vi "niDTS WLAN UTIL to Payload Length.vi"(9 "CH BW":T1, 10 "WLAN Type":T2) -> (2 "Payload Length":i32)   [LabVIEW 2015, in "niDTS WLAN.lvlib"]
uses:
  niDTS WLAN.lvlib
  Includes/niDTS WLAN INC Type.ctl
  Includes/niDTS WLAN INC CH BW.ctl
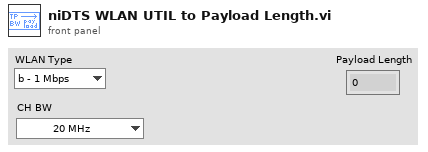
[diagram p1: front panel]
types:
  T1 = typedef "niDTS WLAN.lvlib/niDTS WLAN INC CH BW.ctl" = enum16{"20 MHz", "40 MHz", "80 MHz", "160 MHz"}
  T2 = typedef "niDTS WLAN.lvlib/niDTS WLAN INC Type.ctl" = enum16{"b - 1 Mbps", "b - 2 Mbps", "b - 5.5 Mbps", "b - 11 Mbps", "ag - 6 Mbps", "ag - 9 Mbps", "ag - 12 Mbps", "ag - 18 Mbps", "ag - 24 Mbps", "ag - 36 Mbps", "ag - 48 Mbps", "ag - 54 Mbps", "n - MCS0", "n - MCS1", "n - MCS2", "n - MCS3", "n - MCS4", "n - MCS5", "n - MCS6", "n - MCS7", "n - MCS8", "n - MCS9", "n - MCS10", "n - MCS11", "n - MCS12", "n - MCS13", "n - MCS14", "n - MCS15", "n - MCS16", "n - MCS17", "n - MCS18", "n - MCS19", "n - MCS20", "n - MCS21", "n - MCS22", "n - MCS23", "n - MCS24", "n - MCS25", "n - MCS26", "n - MCS27", "n - MCS28", "n - MCS29", "n - MCS30", "n - MCS31", "ac - MCS0 -1", "ac - MCS1 -1", "ac - MCS2 -1", "ac - MCS3 -1", "ac - MCS4 -1", "ac - MCS5 -1", "ac - MCS6 -1", "ac - MCS7 -1", "ac - MCS8 -1", "ac - MCS9 -1", "ac - MCS0 -2", "ac - MCS1 -2", "ac - MCS2 -2", "ac - MCS3 -2", "ac - MCS4 -2", "ac - MCS5 -2", "ac - MCS6 -2", "ac - MCS7 -2", "ac - MCS8 -2", "ac - MCS9 -2", "ac - MCS0 -3", "ac - MCS1 -3", "ac - MCS2 -3", "ac - MCS3 -3", "ac - MCS4 -3", "ac - MCS5 -3", "ac - MCS6 -3", "ac - MCS7 -3", "ac - MCS8 -3", "ac - MCS9 -3", "ac - MCS0 -4", "ac - MCS1 -4", "ac - MCS2 -4", "ac - MCS3 -4", "ac - MCS4 -4", "ac - MCS5 -4", "ac - MCS6 -4", "ac - MCS7 -4", "ac - MCS8 -4", "ac - MCS9 -4"}
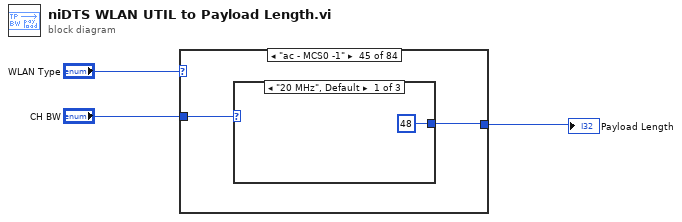
[diagram p0: block diagram]
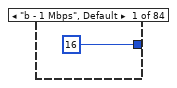
[diagram p2: hidden frame]
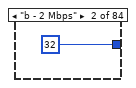
[diagram p3: hidden frame]
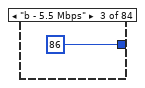
[diagram p4: hidden frame]
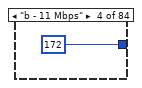
[diagram p5: hidden frame]
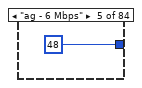
[diagram p6: hidden frame]
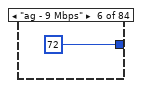
[diagram p7: hidden frame]
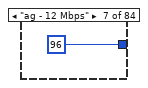
[diagram p8: hidden frame]
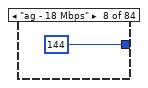
[diagram p9: hidden frame]
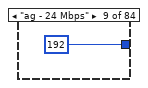
[diagram p10: hidden frame]
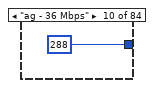
[diagram p11: hidden frame]
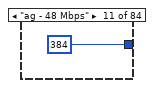
[diagram p12: hidden frame]
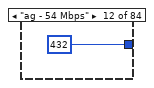
[diagram p13: hidden frame]
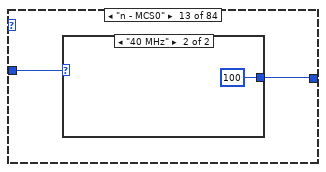
[diagram p14: hidden frame]
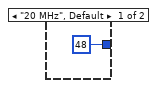
[diagram p15: hidden frame]
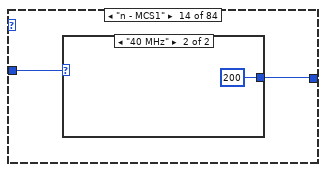
[diagram p16: hidden frame]
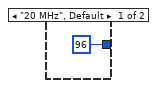
[diagram p17: hidden frame]
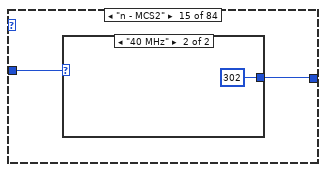
[diagram p18: hidden frame]
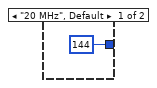
[diagram p19: hidden frame]
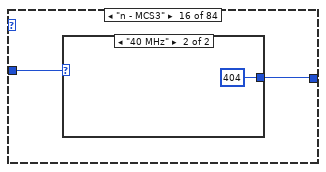
[diagram p20: hidden frame]
diagram:
  n1 = case shown="\"ac - MCS0 -1\"" "WLAN Type" {
    tunnel: [16 ("Payload Length") 32 ("Payload Length") 86 ("Payload Length") 172 ("Payload Length") 48 ("Payload Length") 72 ("Payload Length") 96 ("Payload Length") 144 ("Payload Length") 192 ("Payload Length") 288 ("Payload Length") 384 ("Payload Length") 432 ("Payload Length") w16 w20 w24 w28 w32 w36 w40 w44 w48 w52 w56 w60 w64 w68 w72 w76 w80 w84 w88 w92 w96 w100 w104 w108 w112 w116 w120 w124 w128 w132 w136 w140 w144 w149 w154 w159 w164 w169 w174 w179 w184 w189 w194 w199 w204 w209 w214 w219 w224 w229 w234 w239 w244 w249 w254 w259 w264 w269 w274 w279 w284 w289 w294 w299 w304 w309 w314 w319 w324 w329 w334 w339] -> w1
    tunnel: "CH BW" -> [_ _ _ _ _ _ _ _ _ _ _ _ w17 w21 w25 w29 w33 w37 w41 w45 w49 w53 w57 w61 w65 w69 w73 w77 w81 w85 w89 w93 w97 w101 w105 w109 w113 w117 w121 w125 w129 w133 w137 w141 w145 w150 w155 w160 w165 w170 w175 w180 w185 w190 w195 w200 w205 w210 w215 w220 w225 w230 w235 w240 w245 w250 w255 w260 w265 w270 w275 w280 w285 w290 w295 w300 w305 w310 w315 w320 w325 w330 w335 w340]
    frame "b - 1 Mbps", Default {
    }
    frame "b - 2 Mbps" {
    }
    frame "b - 5.5 Mbps" {
    }
    frame "b - 11 Mbps" {
    }
    frame "ag - 6 Mbps" {
    }
    frame "ag - 9 Mbps" {
    }
    frame "ag - 12 Mbps" {
    }
    frame "ag - 18 Mbps" {
    }
    frame "ag - 24 Mbps" {
    }
    frame "ag - 36 Mbps" {
    }
    frame "ag - 48 Mbps" {
    }
    frame "ag - 54 Mbps" {
    }
    frame "n - MCS0" {
      n2 = case shown="\"40 MHz\"" w17 {
        tunnel: [48 ("Data Length") 100 ("Data Length")] -> w16
        frame "20 MHz", Default {
        }
        frame "40 MHz" {
        }
      }
    }
    frame "n - MCS1" {
      n3 = case shown="\"40 MHz\"" w21 {
        tunnel: [96 ("Data Length") 200 ("Data Length")] -> w20
        frame "20 MHz", Default {
        }
        frame "40 MHz" {
        }
      }
    }
    frame "n - MCS2" {
      n4 = case shown="\"40 MHz\"" w25 {
        tunnel: [144 ("Data Length") 302 ("Data Length")] -> w24
        frame "20 MHz", Default {
        }
        frame "40 MHz" {
        }
      }
    }
    frame "n - MCS3" {
      n5 = case shown="\"40 MHz\"" w29 {
        tunnel: [194 ("Data Length") 404 ("Data Length")] -> w28
        frame "20 MHz", Default {
        }
        frame "40 MHz" {
        }
      }
    }
    frame "n - MCS4" {
      n6 = case shown="\"40 MHz\"" w33 {
        tunnel: [290 ("Data Length") 606 ("Data Length")] -> w32
        frame "20 MHz", Default {
        }
        frame "40 MHz" {
        }
      }
    }
    frame "n - MCS5" {
      n7 = case shown="\"40 MHz\"" w37 {
        tunnel: [388 ("Data Length") 808 ("Data Length")] -> w36
        frame "20 MHz", Default {
        }
        frame "40 MHz" {
        }
      }
    }
    frame "n - MCS6" {
      n8 = case shown="\"40 MHz\"" w41 {
        tunnel: [438 ("Data Length") 910 ("Data Length")] -> w40
        frame "20 MHz", Default {
        }
        frame "40 MHz" {
        }
      }
    }
    frame "n - MCS7" {
      n9 = case shown="\"40 MHz\"" w45 {
        tunnel: [486 ("Data Length") 1010 ("Data Length")] -> w44
        frame "20 MHz", Default {
        }
        frame "40 MHz" {
        }
      }
    }
    frame "n - MCS8" {
      n10 = case shown="\"40 MHz\"" w49 {
        tunnel: [60 ("Data Length") 166 ("Data Length")] -> w48
        frame "20 MHz", Default {
        }
        frame "40 MHz" {
        }
      }
    }
    frame "n - MCS9" {
      n11 = case shown="\"40 MHz\"" w53 {
        tunnel: [160 ("Data Length") 370 ("Data Length")] -> w52
        frame "20 MHz", Default {
        }
        frame "40 MHz" {
        }
      }
    }
    frame "n - MCS10" {
      n12 = case shown="\"40 MHz\"" w57 {
        tunnel: [256 ("Data Length") 572 ("Data Length")] -> w56
        frame "20 MHz", Default {
        }
        frame "40 MHz" {
        }
      }
    }
    frame "n - MCS11" {
      n13 = case shown="\"40 MHz\"" w61 {
        tunnel: [354 ("Data Length") 774 ("Data Length")] -> w60
        frame "20 MHz", Default {
        }
        frame "40 MHz" {
        }
      }
    }
    frame "n - MCS12" {
      n14 = case shown="\"40 MHz\"" w65 {
        tunnel: [550 ("Data Length") 1180 ("Data Length")] -> w64
        frame "20 MHz", Default {
        }
        frame "40 MHz" {
        }
      }
    }
    frame "n - MCS13" {
      n15 = case shown="\"40 MHz\"" w69 {
        tunnel: [744 ("Data Length") 1584 ("Data Length")] -> w68
        frame "20 MHz", Default {
        }
        frame "40 MHz" {
        }
      }
    }
    frame "n - MCS14" {
      n16 = case shown="\"40 MHz\"" w73 {
        tunnel: [842 ("Data Length") 1786 ("Data Length")] -> w72
        frame "20 MHz", Default {
        }
        frame "40 MHz" {
        }
      }
    }
    frame "n - MCS15" {
      n17 = case shown="\"40 MHz\"" w77 {
        tunnel: [940 ("Data Length") 1990 ("Data Length")] -> w76
        frame "20 MHz", Default {
        }
        frame "40 MHz" {
        }
      }
    }
    frame "n - MCS16" {
      n18 = case shown="\"40 MHz\"" w81 {
        tunnel: [110 ("Data Length") 268 ("Data Length")] -> w80
        frame "20 MHz", Default {
        }
        frame "40 MHz" {
        }
      }
    }
    frame "n - MCS17" {
      n19 = case shown="\"40 MHz\"" w85 {
        tunnel: [256 ("Data Length") 572 ("Data Length")] -> w84
        frame "20 MHz", Default {
        }
        frame "40 MHz" {
        }
      }
    }
    frame "n - MCS18" {
      n20 = case shown="\"40 MHz\"" w89 {
        tunnel: [404 ("Data Length") 876 ("Data Length")] -> w88
        frame "20 MHz", Default {
        }
        frame "40 MHz" {
        }
      }
    }
    frame "n - MCS19" {
      n21 = case shown="\"40 MHz\"" w93 {
        tunnel: [550 ("Data Length") 1180 ("Data Length")] -> w92
        frame "20 MHz", Default {
        }
        frame "40 MHz" {
        }
      }
    }
    frame "n - MCS20" {
      n22 = case shown="\"40 MHz\"" w97 {
        tunnel: [842 ("Data Length") 1786 ("Data Length")] -> w96
        frame "20 MHz", Default {
        }
        frame "40 MHz" {
        }
      }
    }
    frame "n - MCS21" {
      n23 = case shown="\"40 MHz\"" w101 {
        tunnel: [1134 ("Data Length") 2394 ("Data Length")] -> w100
        frame "20 MHz", Default {
        }
        frame "40 MHz" {
        }
      }
    }
    frame "n - MCS22" {
      n24 = case shown="\"40 MHz\"" w105 {
        tunnel: [1280 ("Data Length") 2698 ("Data Length")] -> w104
        frame "20 MHz", Default {
        }
        frame "40 MHz" {
        }
      }
    }
    frame "n - MCS23" {
      n25 = case shown="\"40 MHz\"" w109 {
        tunnel: [1426 ("Data Length") 3002 ("Data Length")] -> w108
        frame "20 MHz", Default {
        }
        frame "40 MHz" {
        }
      }
    }
    frame "n - MCS24" {
      n26 = case shown="\"40 MHz\"" w113 {
        tunnel: [160 ("Data Length") 370 ("Data Length")] -> w112
        frame "20 MHz", Default {
        }
        frame "40 MHz" {
        }
      }
    }
    frame "n - MCS25" {
      n27 = case shown="\"40 MHz\"" w117 {
        tunnel: [354 ("Data Length") 774 ("Data Length")] -> w116
        frame "20 MHz", Default {
        }
        frame "40 MHz" {
        }
      }
    }
    frame "n - MCS26" {
      n28 = case shown="\"40 MHz\"" w121 {
        tunnel: [550 ("Data Length") 1180 ("Data Length")] -> w120
        frame "20 MHz", Default {
        }
        frame "40 MHz" {
        }
      }
    }
    frame "n - MCS27" {
      n29 = case shown="\"40 MHz\"" w125 {
        tunnel: [744 ("Data Length") 1584 ("Data Length")] -> w124
        frame "20 MHz", Default {
        }
        frame "40 MHz" {
        }
      }
    }
    frame "n - MCS28" {
      n30 = case shown="\"40 MHz\"" w129 {
        tunnel: [1134 ("Data Length") 2394 ("Data Length")] -> w128
        frame "20 MHz", Default {
        }
        frame "40 MHz" {
        }
      }
    }
    frame "n - MCS29" {
      n31 = case shown="\"40 MHz\"" w133 {
        tunnel: [1524 ("Data Length") 3204 ("Data Length")] -> w132
        frame "20 MHz", Default {
        }
        frame "40 MHz" {
        }
      }
    }
    frame "n - MCS30" {
      n32 = case shown="\"40 MHz\"" w137 {
        tunnel: [1720 ("Data Length") 3608 ("Data Length")] -> w136
        frame "20 MHz", Default {
        }
        frame "40 MHz" {
        }
      }
    }
    frame "n - MCS31" {
      n33 = case shown="\"40 MHz\"" w141 {
        tunnel: [1914 ("Data Length") 4014 ("Data Length")] -> w140
        frame "20 MHz", Default {
        }
        frame "40 MHz" {
        }
      }
    }
    frame "ac - MCS0 -1" {
      n34 = case shown="\"20 MHz\", Default" w145 {
        tunnel: [48 ("Data Length") 100 ("Data Length") 218 ("Data Length")] -> w144
        frame "20 MHz", Default {
        }
        frame "40 MHz" {
        }
        frame "80 MHz" {
        }
      }
    }
    frame "ac - MCS0 -2" {
      n35 = case shown="\"80 MHz\"" w150 {
        tunnel: [52 ("Data Length") 150 ("Data Length") 404 ("Data Length")] -> w149
        frame "20 MHz", Default {
        }
        frame "40 MHz" {
        }
        frame "80 MHz" {
        }
      }
    }
    frame "ac - MCS0 -3" {
      n36 = case shown="\"80 MHz\"" w155 {
        tunnel: [106 ("Data Length") 244 ("Data Length") 620 ("Data Length")] -> w154
        frame "20 MHz", Default {
        }
        frame "40 MHz" {
        }
        frame "80 MHz" {
        }
      }
    }
    frame "ac - MCS0 -4" {
      n37 = case shown="\"80 MHz\"" w160 {
        tunnel: [144 ("Data Length") 340 ("Data Length") 838 ("Data Length")] -> w159
        frame "20 MHz", Default {
        }
        frame "40 MHz" {
        }
        frame "80 MHz" {
        }
      }
    }
    frame "ac - MCS1 -1" {
      n38 = case shown="\"80 MHz\"" w165 {
        tunnel: [96 ("Data Length") 200 ("Data Length") 438 ("Data Length")] -> w164
        frame "20 MHz", Default {
        }
        frame "40 MHz" {
        }
        frame "80 MHz" {
        }
      }
    }
    frame "ac - MCS1 -2" {
      n39 = case shown="\"80 MHz\"" w170 {
        tunnel: [144 ("Data Length") 340 ("Data Length") 838 ("Data Length")] -> w169
        frame "20 MHz", Default {
        }
        frame "40 MHz" {
        }
        frame "80 MHz" {
        }
      }
    }
    frame "ac - MCS1 -3" {
      n40 = case shown="\"80 MHz\"" w175 {
        tunnel: [234 ("Data Length") 568 ("Data Length") 1304 ("Data Length")] -> w174
        frame "20 MHz", Default {
        }
        frame "40 MHz" {
        }
        frame "80 MHz" {
        }
      }
    }
    frame "ac - MCS1 -4" {
      n41 = case shown="\"80 MHz\"" w180 {
        tunnel: [326 ("Data Length") 772 ("Data Length") 1716 ("Data Length")] -> w179
        frame "20 MHz", Default {
        }
        frame "40 MHz" {
        }
        frame "80 MHz" {
        }
      }
    }
    frame "ac - MCS2 -1" {
      n42 = case shown="\"80 MHz\"" w185 {
        tunnel: [144 ("Data Length") 302 ("Data Length") 656 ("Data Length")] -> w184
        frame "20 MHz", Default {
        }
        frame "40 MHz" {
        }
        frame "80 MHz" {
        }
      }
    }
    frame "ac - MCS2 -2" {
      n43 = case shown="\"80 MHz\"" w190 {
        tunnel: [234 ("Data Length") 528 ("Data Length") 1302 ("Data Length")] -> w189
        frame "20 MHz", Default {
        }
        frame "40 MHz" {
        }
        frame "80 MHz" {
        }
      }
    }
    frame "ac - MCS2 -3" {
      n44 = case shown="\"80 MHz\"" w195 {
        tunnel: [410 ("Data Length") 920 ("Data Length") 1936 ("Data Length")] -> w194
        frame "20 MHz", Default {
        }
        frame "40 MHz" {
        }
        frame "80 MHz" {
        }
      }
    }
    frame "ac - MCS2 -4" {
      n45 = case shown="\"80 MHz\"" w200 {
        tunnel: [508 ("Data Length") 1220 ("Data Length") 2620 ("Data Length")] -> w199
        frame "20 MHz", Default {
        }
        frame "40 MHz" {
        }
        frame "80 MHz" {
        }
      }
    }
    frame "ac - MCS3 -1" {
      n46 = case shown="\"80 MHz\"" w205 {
        tunnel: [194 ("Data Length") 404 ("Data Length") 876 ("Data Length")] -> w204
        frame "20 MHz", Default {
        }
        frame "40 MHz" {
        }
        frame "80 MHz" {
        }
      }
    }
    frame "ac - MCS3 -2" {
      n47 = case shown="\"80 MHz\"" w210 {
        tunnel: [326 ("Data Length") 772 ("Data Length") 1716 ("Data Length")] -> w209
        frame "20 MHz", Default {
        }
        frame "40 MHz" {
        }
        frame "80 MHz" {
        }
      }
    }
    frame "ac - MCS3 -3" {
      n48 = case shown="\"80 MHz\"" w215 {
        tunnel: [546 ("Data Length") 1202 ("Data Length") 2620 ("Data Length")] -> w214
        frame "20 MHz", Default {
        }
        frame "40 MHz" {
          (unwired) 1176 ("Data Length")
        }
        frame "80 MHz" {
        }
      }
    }
    frame "ac - MCS3 -4" {
      n49 = case shown="\"80 MHz\"" w220 {
        tunnel: [742 ("Data Length") 1620 ("Data Length") 3472 ("Data Length")] -> w219
        frame "20 MHz", Default {
        }
        frame "40 MHz" {
        }
        frame "80 MHz" {
        }
      }
    }
    frame "ac - MCS4 -1" {
      n50 = case shown="\"80 MHz\"" w225 {
        tunnel: [290 ("Data Length") 606 ("Data Length") 1314 ("Data Length")] -> w224
        frame "20 MHz", Default {
        }
        frame "40 MHz" {
        }
        frame "80 MHz" {
        }
      }
    }
    frame "ac - MCS4 -2" {
      n51 = case shown="\"80 MHz\"" w230 {
        tunnel: [508 ("Data Length") 1220 ("Data Length") 2620 ("Data Length")] -> w229
        frame "20 MHz", Default {
        }
        frame "40 MHz" {
        }
        frame "80 MHz" {
        }
      }
    }
    frame "ac - MCS4 -3" {
      n52 = case shown="\"80 MHz\"" w235 {
        tunnel: [838 ("Data Length") 1820 ("Data Length") 3910 ("Data Length")] -> w234
        frame "20 MHz", Default {
        }
        frame "40 MHz" {
        }
        frame "80 MHz" {
        }
      }
    }
    frame "ac - MCS4 -4" {
      n53 = case shown="\"80 MHz\"" w240 {
        tunnel: [1132 ("Data Length") 2420 ("Data Length") 5226 ("Data Length")] -> w239
        frame "20 MHz", Default {
        }
        frame "40 MHz" {
        }
        frame "80 MHz" {
        }
      }
    }
    frame "ac - MCS5 -1" {
      n54 = case shown="\"80 MHz\"" w245 {
        tunnel: [388 ("Data Length") 808 ("Data Length") 1754 ("Data Length")] -> w244
        frame "20 MHz", Default {
        }
        frame "40 MHz" {
        }
        frame "80 MHz" {
        }
      }
    }
    frame "ac - MCS5 -2" {
      n55 = case shown="\"80 MHz\"" w250 {
        tunnel: [742 ("Data Length") 1610 ("Data Length") 3472 ("Data Length")] -> w249
        frame "20 MHz", Default {
        }
        frame "40 MHz" {
        }
        frame "80 MHz" {
        }
      }
    }
    frame "ac - MCS5 -3" {
      n56 = case shown="\"80 MHz\"" w255 {
        tunnel: [1132 ("Data Length") 2420 ("Data Length") 5226 ("Data Length")] -> w254
        frame "20 MHz", Default {
        }
        frame "40 MHz" {
        }
        frame "80 MHz" {
        }
      }
    }
    frame "ac - MCS5 -4" {
      n57 = case shown="\"80 MHz\"" w260 {
        tunnel: [1522 ("Data Length") 3302 ("Data Length") 7020 ("Data Length")] -> w259
        frame "20 MHz", Default {
        }
        frame "40 MHz" {
        }
        frame "80 MHz" {
        }
      }
    }
    frame "ac - MCS6 -1" {
      n58 = case shown="\"80 MHz\"" w265 {
        tunnel: [438 ("Data Length") 910 ("Data Length") 1972 ("Data Length")] -> w264
        frame "20 MHz", Default {
        }
        frame "40 MHz" {
        }
        frame "80 MHz" {
        }
      }
    }
    frame "ac - MCS6 -2" {
      n59 = case shown="\"80 MHz\"" w270 {
        tunnel: [838 ("Data Length") 1820 ("Data Length") 3910 ("Data Length")] -> w269
        frame "20 MHz", Default {
        }
        frame "40 MHz" {
        }
        frame "80 MHz" {
        }
      }
    }
    frame "ac - MCS6 -3" {
      n60 = case shown="\"80 MHz\"" w275 {
        tunnel: [1320 ("Data Length") 2720 ("Data Length") 0 ("Data Length")] -> w274
        frame "20 MHz", Default {
        }
        frame "40 MHz" {
        }
        frame "80 MHz" {
          # "This is not allowed"
        }
      }
    }
    frame "ac - MCS6 -4" {
      n61 = case shown="\"80 MHz\"" w280 {
        tunnel: [1716 ("Data Length") 3606 ("Data Length") 7858 ("Data Length")] -> w279
        frame "20 MHz", Default {
        }
        frame "40 MHz" {
        }
        frame "80 MHz" {
        }
      }
    }
    frame "ac - MCS7 -1" {
      n62 = case shown="\"80 MHz\"" w285 {
        tunnel: [486 ("Data Length") 1010 ("Data Length") 2192 ("Data Length")] -> w284
        frame "20 MHz", Default {
        }
        frame "40 MHz" {
        }
        frame "80 MHz" {
        }
      }
    }
    frame "ac - MCS7 -2" {
      n63 = case shown="\"80 MHz\"" w290 {
        tunnel: [936 ("Data Length") 2020 ("Data Length") 4348 ("Data Length")] -> w289
        frame "20 MHz", Default {
        }
        frame "40 MHz" {
        }
        frame "80 MHz" {
        }
      }
    }
    frame "ac - MCS7 -3" {
      n64 = case shown="\"80 MHz\"" w295 {
        tunnel: [1424 ("Data Length") 3020 ("Data Length") 6542 ("Data Length")] -> w294
        frame "20 MHz", Default {
        }
        frame "40 MHz" {
        }
        frame "80 MHz" {
        }
      }
    }
    frame "ac - MCS7 -4" {
      n65 = case shown="\"80 MHz\"" w300 {
        tunnel: [1912 ("Data Length") 4012 ("Data Length") 8736 ("Data Length")] -> w299
        frame "20 MHz", Default {
        }
        frame "40 MHz" {
        }
        frame "80 MHz" {
        }
      }
    }
    frame "ac - MCS8 -1" {
      n66 = case shown="\"80 MHz\"" w305 {
        tunnel: [584 ("Data Length") 1214 ("Data Length") 2630 ("Data Length")] -> w304
        frame "20 MHz", Default {
        }
        frame "40 MHz" {
        }
        frame "80 MHz" {
        }
      }
    }
    frame "ac - MCS8 -2" {
      n67 = case shown="\"80 MHz\"" w310 {
        tunnel: [1132 ("Data Length") 2500 ("Data Length") 5226 ("Data Length")] -> w309
        frame "20 MHz", Default {
        }
        frame "40 MHz" {
        }
        frame "80 MHz" {
        }
      }
    }
    frame "ac - MCS8 -3" {
      n68 = case shown="\"80 MHz\"" w315 {
        tunnel: [1716 ("Data Length") 3606 ("Data Length") 7858 ("Data Length")] -> w314
        frame "20 MHz", Default {
        }
        frame "40 MHz" {
        }
        frame "80 MHz" {
        }
      }
    }
    frame "ac - MCS8 -4" {
      n69 = case shown="\"80 MHz\"" w320 {
        tunnel: [2302 ("Data Length") 4822 ("Data Length") 10600 ("Data Length")] -> w319
        frame "20 MHz", Default {
        }
        frame "40 MHz" {
        }
        frame "80 MHz" {
          (unwired) 10492 ("Data Length")
          # "15 symbols"
        }
      }
    }
    frame "ac - MCS9 -1" {
      n70 = case shown="\"80 MHz\"" w325 {
        tunnel: [584 ("Data Length") 1348 ("Data Length") 2924 ("Data Length")] -> w324
        frame "20 MHz", Default {
          # "undefined"
        }
        frame "40 MHz" {
        }
        frame "80 MHz" {
        }
      }
    }
    frame "ac - MCS9 -2" {
      n71 = case shown="\"80 MHz\"" w330 {
        tunnel: [0 ("Data Length") 2662 ("Data Length") 5812 ("Data Length")] -> w329
        frame "20 MHz", Default {
          # "undefined"
        }
        frame "40 MHz" {
        }
        frame "80 MHz" {
        }
      }
    }
    frame "ac - MCS9 -3" {
      n72 = case shown="\"80 MHz\"" w335 {
        tunnel: [0 ("Data Length") 4012 ("Data Length") 8739 ("Data Length")] -> w334
        frame "20 MHz", Default {
          # "undefined"
        }
        frame "40 MHz" {
        }
        frame "80 MHz" {
        }
      }
    }
    frame "ac - MCS9 -4" {
      n73 = case shown="\"80 MHz\"" w340 {
        tunnel: [0 ("Data Length") 5362 ("Data Length") 11662 ("Data Length")] -> w339
        frame "20 MHz", Default {
          # "undefined"
        }
        frame "40 MHz" {
        }
        frame "80 MHz" {
        }
      }
    }
  }
  "Payload Length" <- w1
